vi "FlatToRichrfcontrol_RFRequest.vi"(5 "OutputClusterType":T1, 11 "InputCluster":T2) -> (3 "OutputCluster":T1)   [LabVIEW 2024, in "FlexSDR_gRPC_client.lvlib"]
uses:
  rfcontrol_RFRequest_Flat.ctl
  rfcontrol_RFRequest.ctl
  FlexSDR_gRPC_client.lvlib
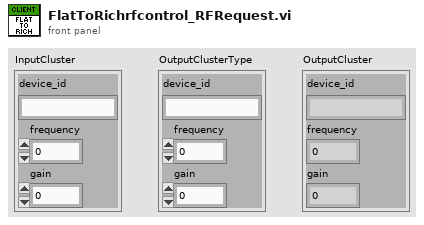
[diagram p1: front panel]
types:
  T1 = typedef "FlexSDR_gRPC_client.lvlib/rfcontrol_RFRequest.ctl" = cluster{"device_id":string, "frequency":dbl, "gain":dbl}
  T2 = typedef "FlexSDR_gRPC_client.lvlib/rfcontrol_RFRequest_Flat.ctl" = cluster{"device_id":string, "frequency":dbl, "gain":dbl}
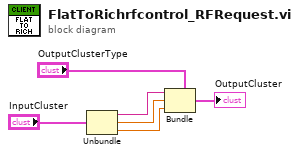
[diagram p0: block diagram]
diagram:
  n1 = Unbundle "Unbundle"("InputCluster") -> ("device_id"=w3:string, "frequency"=w2:dbl, "gain"=w1:dbl)
  n2 = Bundle "Bundle"(cluster="OutputClusterType", "device_id"=w3, "frequency"=w2, "gain"=w1) -> (→"OutputCluster":T1)
